vi "_ql2proto_parser.vi"() -> ()   [LabVIEW 2017]
panel:
  out "ids":u32[](array[numeric])
  in  "ring":u8(ring) items=["SUCCESS_ATOM", "SUCCESS_SEQUENCE", "SUCCESS_PARTIAL", "WAIT_COMPLETE", "SERVER_INFO", "CLIENT_ERROR", "COMPILE_ERROR", "RUNTIME_ERROR"]
  in  "String":string
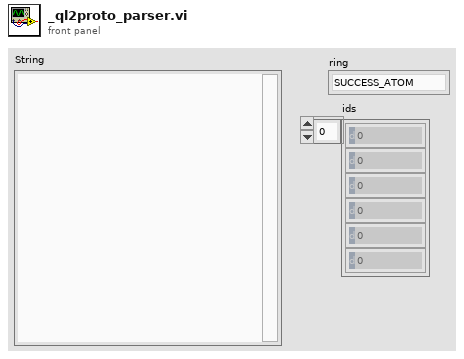
[diagram p1: front panel]
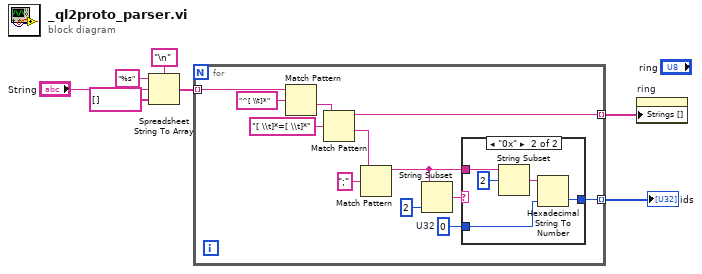
[diagram p0: block diagram]
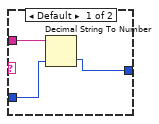
[diagram p2: hidden frame]
diagram:
  n1 = Spreadsheet String To Array(delimiter (Tab)="\n", format string="%s", spreadsheet string="String", array type (2D Dbl)=string[] []) -> (array=w3:string[])
  n2 = for {
    tunnel: w3 -> [w19] mode=indexing
    tunnel: [w15] -> w2 mode=indexing
    tunnel: [w8] -> w1 mode=indexing
    w9 = u32 0  # U32
    n3 = Match Pattern(string=w19, regular expression="^[ \\t]*") -> (after substring=w17:string)  [unwired: 1 in, 3 out]
    n4 = Match Pattern(string=w17, regular expression="[ \\t]*=[ \\t]*") -> (before substring=w15:string, after substring=w13:string)  [unwired: 1 in, 2 out]
    n5 = Match Pattern(string=w13, regular expression=";") -> (before substring=w10:string)  [unwired: 1 in, 3 out]
    n6 = String Subset(string=w10, length (rest)=2 ("length (rest)")) -> (substring=w11:string)  [unwired: 1 in]
    n7 = case shown="\"0x\"" w11 {
      tunnel: w10 -> [w22 w27]
      tunnel: w9 -> [w21 w24]
      tunnel: [w20 w23] -> w8
      frame Default {
        n8 = Decimal String To Number(string=w22, default (0L)=w21) -> (number=w20:u32)  [unwired: 1 in, 1 out]
      }
      frame "0x" {
        n9 = String Subset(string=w27, offset (0)=2) -> (substring=w25:string)  [unwired: 1 in]
        n10 = Hexadecimal String To Number(string=w25, default (0uL)=w24) -> (number=w23:u32)  [unwired: 1 in, 1 out]
      }
    }
  }
  "ids" <- w1
  n11 = property on="ring" class="Ring (strict)"("Strings []"=w2) -> ()  [unwired: 2 in, 2 out]
